vi "CheckVisInMemory.vi"() -> ()   [LabVIEW 2015]
panel:
  out "Array":path[](array[path])
  in  "Move?":bool
  out "Application:All VIs Not In Memory":string[](array[string])
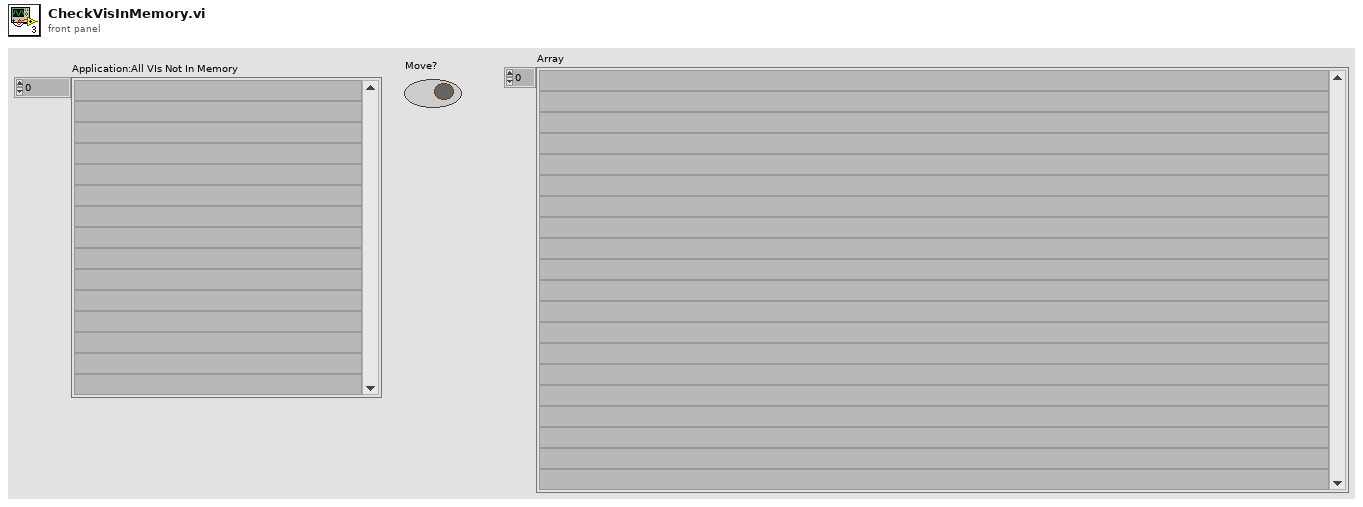
[diagram p1: front panel]
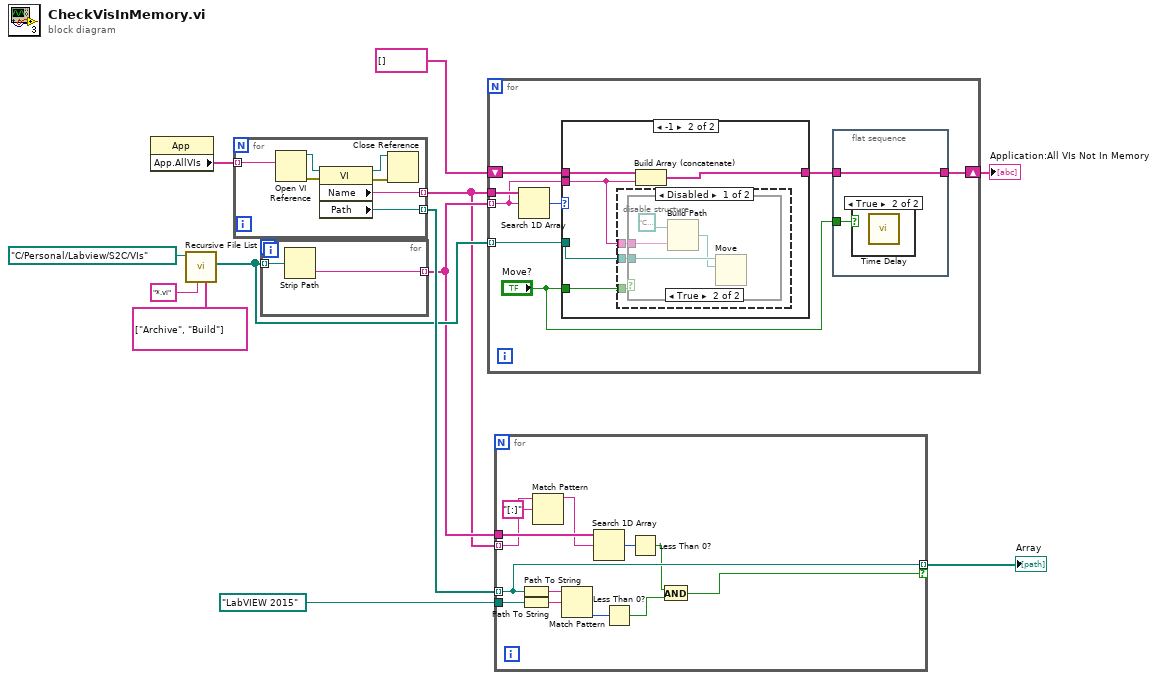
[diagram p0: block diagram]
diagram:
  n1 = property class="App"() -> ("App.AllVIs"=w12:string[])  [unwired: 2 in, 2 out]
  n2 = call <vilib>:"Recursive File List.vi"("Folders to Exclude"=string[] ["Archive", "Build"], "pattern"="*.vi", "Folder Path"=path "C:/Personal/Labview/S2C/VIs") -> ("All Files in Dir"=w5:path[])  [unwired: 4 in, 4 out]
  n3 = for {
    tunnel: w12 -> [w13] mode=indexing
    tunnel: [w15] -> w1 mode=indexing
    tunnel: [w14] -> w6 mode=indexing
    n4 = Open VI Reference(vi path=w13) -> (vi reference=w18:refnum<vi>, error out=w19:errorcluster)  [unwired: 5 in]
    n5 = property class="VI"(reference=w18, error in=w19) -> (reference out=w16:refnum<vi>, error out=w17:errorcluster, "Name"=w15:string, "Path"=w14:path)
    n6 = Close Reference(reference=w16, error in (no error)=w17) -> ()  [unwired: 1 out]
  }
  n7 = for {
    tunnel: w5 -> [w21] mode=indexing
    tunnel: [w20] -> w2 mode=indexing
    n8 = Strip Path(path=w21) -> (name=w20:string)  [unwired: 1 out]
  }
  n9 = for {
    tunnel: w1 -> [w29]
    tunnel: w2 -> [w26] mode=indexing
    shift-right: [w23] -> w7
    shift-left: string[] [] ("Application:All VIs In Memory") -> [w27]
    tunnel: w5 -> [w25] mode=indexing
    n10 = Search 1D Array(1D array=w29, element=w26) -> (index of element=w28:i32)  [unwired: 1 in]
    n11 = case shown="-1" w28 {
      tunnel: w27 -> [w32 w37]
      tunnel: w26 -> [_ w34]
      tunnel: [w32 w36] -> w24
      tunnel: w25 -> [_ w35]
      tunnel: "Move?" -> [_ w33]
      frame 0, Default {
      }
      frame -1 {
        n12 = disable-structure shown="Disabled" {
          disable-tunnel: w35 -> [w40 _]
          disable-tunnel: w34 -> [w39 _]
          disable-tunnel: w33 -> [w38 _]
          frame Disabled {
            n13 = case shown="True" w38 {
              tunnel: w40 -> [_ w44]
              tunnel: w39 -> [_ w43]
              frame False {
              }
              frame True {
                n14 = Build Path(base path=path "C:/Medtronic/Labview/Dissector Tester/Archive" ("target path (use dialog)"), name or relative path=w43) -> (appended path=w41:path)
                n15 = Move(source path=w44, 10:w41) -> ()  [unwired: 3 in, 3 out]
              }
            }
          }
          frame Enabled {
          }
        }
        n16 = Build Array (concatenate)(w37, w34) -> (w36:string[])
      }
    }
    n17 = flat-sequence {
      tunnel: w24 -> [w31]
      tunnel: [w31] -> w23
      tunnel: "Move?" -> [w30]
      frame #0 {
        n18 = case shown="True" w30 {
          frame False {
          }
          frame True {
            n19 = call "Time Delay"() -> ()  [unwired: 11 in, 1 out]
          }
        }
      }
    }
  }
  "Application:All VIs Not In Memory" <- w7
  n20 = for {
    tunnel: w6 -> [w52] mode=indexing
    tunnel: w2 -> [w57]
    tunnel: [w52] -> w4 mode=indexing if=w48
    tunnel: path "LabVIEW 2015" ("Folder Path") -> [w54]
    tunnel: w1 -> [w47] mode=indexing
    n21 = Path To String(path=w52) -> (string=w53:string)
    n22 = Path To String(path=w54) -> (string=w55:string)
    n23 = Match Pattern(string=w47, regular expression="[:]") -> (before substring=w45:string)  [unwired: 1 in, 3 out]
    n24 = Match Pattern(string=w53, regular expression=w55) -> (offset past match=w51:i32)  [unwired: 1 in, 3 out]
    n25 = Search 1D Array(1D array=w57, element=w45) -> (index of element=w56:i32)  [unwired: 1 in]
    n26 = Less Than 0?(x=w51) -> (x < 0?=w50:bool)
    n27 = Less Than 0?(x=w56) -> (x < 0?=w49:bool)
    n28 = And(x=w49, y=w50) -> (x .and. y?=w48:bool)
  }
  "Array" <- w4
